vi "Pre-Build Custom Action.vi"(10 "Variant":variant) -> (0 "error out":errorcluster)   [LabVIEW 2017]
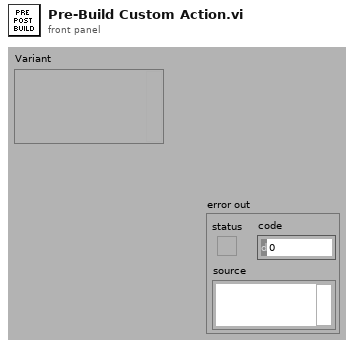
[diagram p1: front panel]
types:
  T1 = cluster{"CreateSnippet":bool, "SnippetHeader":string, "EmbeddedHeader":string, "HeaderColor":u32, "Version":string}
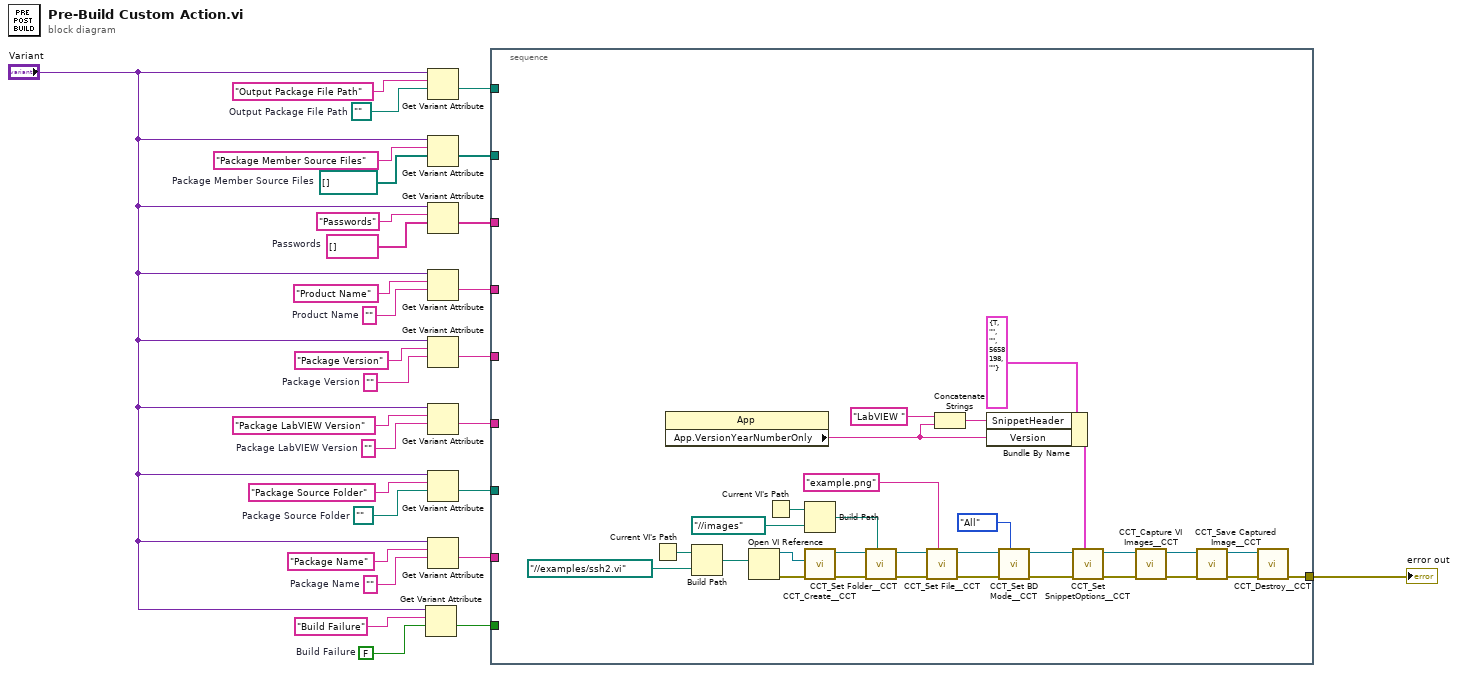
[diagram p0: block diagram]
diagram:
  w4 = FALSE  # Build Failure
  w14 = path ""  # Package Source Folder
  w15 = ""  # Package Name
  w18 = ""  # Package LabVIEW Version
  w20 = ""  # Package Version
  w22 = ""  # Product Name
  w24 = string[] []  # Passwords
  w26 = path[] []  # Package Member Source Files
  w28 = path ""  # Output Package File Path
  n1 = Get Variant Attribute(Variant="Variant", name="Build Failure", default value (empty Variant)=w4) -> (value=w2:bool)  [unwired: 1 in, 3 out]
  n2 = Get Variant Attribute(Variant="Variant", name="Output Package File Path", default value (empty Variant)=w28) -> (value=w13:path)  [unwired: 1 in, 3 out]
  n3 = Get Variant Attribute(Variant="Variant", name="Package Member Source Files", default value (empty Variant)=w26) -> (value=w12:path[])  [unwired: 1 in, 3 out]
  n4 = Get Variant Attribute(Variant="Variant", name="Passwords", default value (empty Variant)=w24) -> (value=w11:string[])  [unwired: 1 in, 3 out]
  n5 = Get Variant Attribute(Variant="Variant", name="Product Name", default value (empty Variant)=w22) -> (value=w10:string)  [unwired: 1 in, 3 out]
  n6 = Get Variant Attribute(Variant="Variant", name="Package Version", default value (empty Variant)=w20) -> (value=w9:string)  [unwired: 1 in, 3 out]
  n7 = Get Variant Attribute(Variant="Variant", name="Package LabVIEW Version", default value (empty Variant)=w18) -> (value=w8:string)  [unwired: 1 in, 3 out]
  n8 = Get Variant Attribute(Variant="Variant", name="Package Source Folder", default value (empty Variant)=w14) -> (value=w7:path)  [unwired: 1 in, 3 out]
  n9 = Get Variant Attribute(Variant="Variant", name="Package Name", default value (empty Variant)=w15) -> (value=w6:string)  [unwired: 1 in, 3 out]
  n10 = stacked-sequence {
    tunnel: w13 -> [_]
    tunnel: w12 -> [_]
    tunnel: w11 -> [_]
    tunnel: w10 -> [_]
    tunnel: w9 -> [_]
    tunnel: w8 -> [_]
    tunnel: w7 -> [_]
    tunnel: w6 -> [_]
    tunnel: w2 -> [_]
    tunnel: [w44] -> w1
    frame #0 {
      n11 = Current VI's Path() -> (path=w47:path)
      n12 = property class="App"() -> ("App.VersionYearNumberOnly"=w32:string)  [unwired: 2 in, 2 out]
      n13 = Build Path(base path=w47, name or relative path=path "../../examples/ssh2.vi") -> (appended path=w45:path)
      n14 = Open VI Reference(vi path=w45) -> (vi reference=w43:refnum<vi>, error out=w34:errorcluster)  [unwired: 5 in]
      n15 = Current VI's Path() -> (path=w48:path)
      n16 = Build Path(base path=w48, name or relative path=path "../../images") -> (appended path=w50:path)
      n17 = call <vilib>:"CCT_Create__CCT.vi"("error in (no error)"=w34, "VI to capture"=w43) -> ("error out"=w58:errorcluster, "New CCT Instance"=w59:refnum<k1>)  [unwired: 8 in]
      n18 = call <vilib>:"CCT_Set Folder__CCT.vi"("Target Folder"=w50, "error in (no error)"=w58, "reference"=w59) -> ("error out"=w56:errorcluster, "duplicate reference"=w57:refnum<k1>)  [unwired: 7 in]
      n19 = call <vilib>:"CCT_Set File__CCT.vi"("Image File Name"="example.png", "error in (no error)"=w56, "reference"=w57) -> ("error out"=w41:errorcluster, "duplicate reference"=w40:refnum<k1>)  [unwired: 7 in]
      n20 = Concatenate Strings("LabVIEW " ("string"), w32) -> (w30:string)
      n21 = Bundle By Name(cluster=T1 {"CreateSnippet"=TRUE, "SnippetHeader"="", "EmbeddedHeader"="", "HeaderColor"=5658198, "Version"=""} ("Snippet Header"), "SnippetHeader"=w30, "Version"=w32) -> (w33:T1)
      n22 = call <vilib>:"CCT_Set BD Mode__CCT.vi"("BD Mode"=enum16{"No", "Selected", "Visible", "All"}."All", "error in (no error)"=w41, "reference"=w40) -> ("error out"=w36:errorcluster, "duplicate reference"=w38:refnum<k1>)  [unwired: 7 in]
      n23 = call <vilib>:"CCT_Set SnippetOptions__CCT.vi"("Snippet Header"=w33, "error in (no error)"=w36, "reference"=w38) -> ("error out"=w35:errorcluster, "duplicate reference"=w37:refnum<k1>)  [unwired: 7 in]
      n24 = call <vilib>:"CCT_Capture VI Images__CCT.vi"("error in (no error)"=w35, "reference"=w37) -> ("error out"=w54:errorcluster, "duplicate reference"=w55:refnum<k1>)  [unwired: 6 in, 2 out]
      n25 = call <vilib>:"CCT_Save Captured Image__CCT.vi"("error in (no error)"=w54, "reference"=w55) -> ("error out"=w52:errorcluster, "duplicate reference"=w53:refnum<k1>)  [unwired: 7 in, 1 out]
      n26 = call <vilib>:"CCT_Destroy__CCT.vi"("error in (no error)"=w52, "reference"=w53) -> ("error out"=w44:errorcluster)  [unwired: 9 in]
    }
  }
  "error out" <- w1
